vi "pyonpyon2.vi"() -> ()   [LabVIEW 2013]
uses:
  impl/pp2_CTL_SessionInfo.ctl
  impl/pp2_CTL_StateInfo.ctl
  impl/pp2_CTL_State.ctl
  impl/pp2_Trial.ctl
  impl/pp2_CTL_TrialType.ctl
  labolabo2/waveforms/WFTypes.ctl
  impl/pp2_CTL_SessionParamDynamic.ctl
  impl/pp2_CTL_DaqConfig.ctl
  <vilib>/userdefined/High Color/IMAQdx.ctl
  <vilib>/sound2/lvsound2.llb/Sound Output Task ID.ctl
  impl/pp2_CTL_Trial.ctl
  labolabo2/array/impl/NullArray_I.vi
  <vilib>/Utility/file.llb/Read From Spreadsheet File (string).vi
  <vilib>/Utility/file.llb/Write To Spreadsheet File (string).vi
  labolabo2/array/impl/ArrayFirst_S.vi
panel:
  in  "Trial Types Control":enum32{"Trial Types Control"}(tab)
  out "Trial Types File Path":path
  in  "Save Trial Types":bool
  in  "Load Trial Types":bool
  out "Trial Types Valid":bool=TRUE
  in  "Trial Types":T1[](array[typedef])=[{"Trial Type Number"=1, "Trial Type"=enum."GO", "Trial Weight"=1, "Shock (mA)"=-1.0, "Duration (ms)"=250.0, "Sound Type"=enum."04 FM Sweep", "Stim P1"=2000.0, "Stim P2"=4000.0, "Stim P3"=0.0, "Stim P4"=0.0}, {"Trial Type Number"=2, "Trial Type"=enum."NOGO", "Trial Weight"=1, "Shock (mA)"=-1.0, "Duration (ms)"=250.0, "Sound Type"=enum."04 FM Sweep", "Stim P1"=4000.0, "Stim P2"=2000.0, "Stim P3"=0.0, "Stim P4"=0.0}] {"Shock (mA)" min=-1.0 max=5.0; "Trial Weight" step=1; "Duration (ms)" min=0.0 max=1.0; "Trial Type Number" min=1 step=1}
  in  "Session List Control":enum32{"Session List Control"}(tab)
  out "Session List File Path":path=path "E:/Data/SPP.Coulb1/SPP027/ppSessList.141015.1622.tsv"
  in  "Load Session List":bool
  in  "Save Session List":bool
  in  "Generate Session List":bool
  in  "Total Trials":i32=60 min=3 step=1
  in  "Pseudo-Gellerman Start":i32=2 min=2
  out "Session List Valid":bool=TRUE
  out "Session list display":string[][](table)
  in  "Session List Hidden":u8[](array[numeric]) min=1 step=1
  in  "Daq config":T4={"Sound AO"="Dev2/ao0", "Shock intesity AO"="Dev2/ao1", "Code_LED DO"="Dev2/port1:2", "Switch DI"="Dev2/port0/line0:1", "Webcam"="cam9", "Sound AO task"="", "Sound card task"=0, "Shock intensity AO task"="", "Code_LED DO task"="", "Switch DI task"="", "AO <=> Sound card"=FALSE, "Sound card"=0, "sample rate"=8000.0, "Variable shock"=FALSE, "Webcam on"=TRUE, "Tone gate PFI"="/Dev2/PFI1", "Waveform memo"={"t0"=timestamp(0 s since 1904-01-01), "dt"=1.0, "Y"=[]}} {"sample rate" min=8000.0; "Sound card task" format="%.0x"}
  out "Image":T7(plugin-control)
  in  "Session param (dynamic)":T8={"Def M shock (mA)"=400.0, "Def F shock (mA)"=0.0, "Def M shock +/-"=4, "Def F shock +/-"=4} {"Def F shock +/-" min=0 step=1; "Def M shock +/-" min=0 step=1}
  in  "stop":bool
  in  "Pause":bool
  out "State info":T9={"Curr  tr"=0, "Curr (ms)"=0, "Cum (ms)"=0, "Run loop diff"=0, "Tone countdown (ms)"=0, "Countdown (ms)"=0, "Curr State"=enum."0 NULL", "Prev State"=enum."1 Habituation", "Null"=FALSE, "Sw"=FALSE, "Tone\nGate"=FALSE, "Stim"=FALSE, "Current DAQ DO Int"=0, "Current Loaded Trial"={"Trial Type Number"=1, "Trial Type"=enum."GO", "Trial Weight"=100, "Shock (mA)"=0.3, "Duration (ms)"=0.25, "Sound Type"=enum."04 FM Sweep", "Stim P1"=4000.0, "Stim P2"=0.0, "Stim P3"=0.0, "Stim P4"=2000.0}, "Next Trial (for display purposes)"={"Trial Type Number"=1, "Trial Type"=enum."GO", "Trial Weight"=100, "Shock (mA)"=0.3, "Duration (ms)"=0.25, "Sound Type"=enum."04 FM Sweep", "Stim P1"=4000.0, "Stim P2"=0.0, "Stim P3"=0.0, "Stim P4"=2000.0}, "Total trials memo"=0, "State start cum memo (ms)"=0, "Last dur jump time memo (ms)"=0, "Last dur shock time memo (ms)"=0, "Tone repeat memo"=0, "Webcam on"=FALSE, "Webcam recording"=TRUE} {"Current DAQ DO Int" format="%b"; "Next Trial (for display purposes)"."Shock (mA)" min=-1.0 max=5.0; "Next Trial (for display purposes)"."Trial Weight" step=1; "Next Trial (for display purposes)"."Duration (ms)" min=0.0 max=1.0; "Next Trial (for display purposes)"."Trial Type Number" min=1 step=1; "Current Loaded Trial"."Shock (mA)" min=-1.0 max=5.0; "Current Loaded Trial"."Trial Weight" step=1; "Current Loaded Trial"."Duration (ms)" min=0.0 max=1.0; "Current Loaded Trial"."Trial Type Number" min=1 step=1}
  in  "Session parameters":T11={"Log File Directory Root"=path "C:/test", "Habit tr0 (s)"=180, "ITI max\n(s)"=25, "ITI min\n(s)"=15, "Tone repeat (ms)"=0, "Jump time\n(s)"=4, "Subject Name"="SPP030", "Run"=FALSE, "Start trial"=0, "Stay \n(s)"=5, "Log File Directory"=path "", "Shock \ndur (s)"=6, "Pre click \n(V)"=1.0, "Click\ndel (s)"=6} {"Click\ndel (s)" min=0 step=1; "Pre click \n(V)" min=0.0 step=1.0; "Shock \ndur (s)" min=0 step=1; "Stay \n(s)" min=0 step=1; "Start trial" step=1; "Jump time\n(s)" min=0 step=1; "Tone repeat (ms)" min=0 step=1; "ITI min\n(s)" min=0 step=1; "ITI max\n(s)" min=0 step=1; "Habit tr0 (s)" min=0 step=1}
  out "Runtime Errors":errorcluster={"status"=FALSE, "code"=-200552, "source"=""}
  in  "Refresh":bool
  out "Session info":T12
  # "Pyonpyon Labview  v2.5 (2014.12 KT) ktakagak@lin-magdeburg.de)"
  # "Code"
  # "Type"
  # "Dur (ms)"
  # "P 1"
  # "P 2"
  # "P 3"
  # "P 4"
  # "Weight"
  # "Shock"
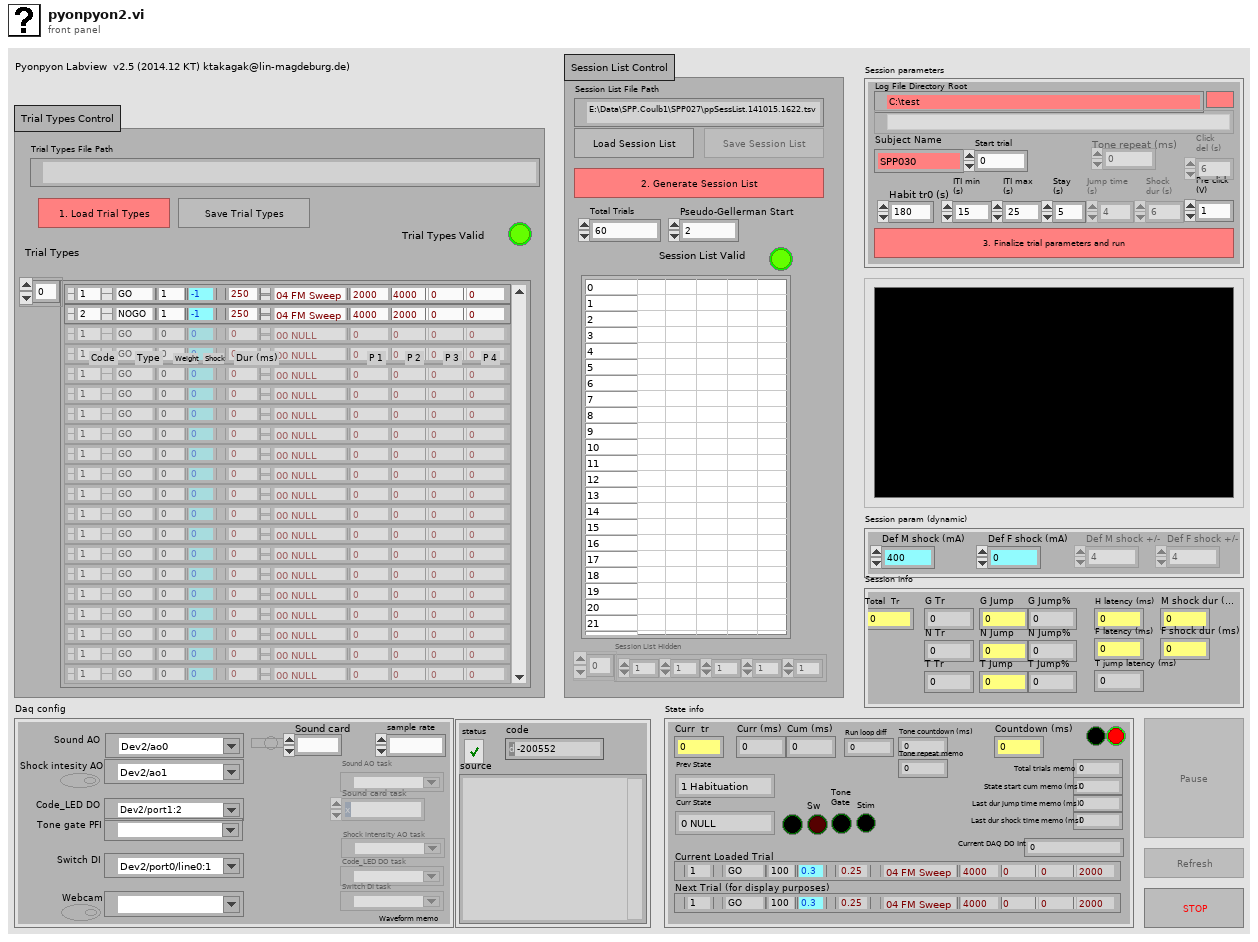
[diagram p1: front panel]
types:
  T1 = typedef "pp2_Trial.ctl" = cluster{"Trial Type Number":u8, "Trial Type":T2, "Trial Weight":u32, "Shock (mA)":dbl, "Duration (ms)":dbl, "Sound Type":T3, "Stim P1":dbl, "Stim P2":dbl, "Stim P3":dbl, "Stim P4":dbl}
  T2 = typedef "pp2_CTL_TrialType.ctl" = enum16{"OFF", "GO", "NOGO", "TEST"}
  T3 = typedef "WFTypes.ctl" = enum16{"00 NULL", "01 DC", "02 Noise", "03 Pure Tone", "04 FM Sweep"}
  T4 = typedef "pp2_CTL_DaqConfig.ctl" = cluster{"Sound AO":tag, "Shock intesity AO":tag, "Code_LED DO":tag, "Switch DI":tag, "Webcam":T5, "Sound AO task":refnum<k21>, "Sound card task":T6, "Shock intensity AO task":refnum<k21>, "Code_LED DO task":refnum<k21>, "Switch DI task":refnum<k21>, "AO <=> Sound card":bool, "Sound card":u32, "sample rate":dbl, "Variable shock":bool, "Webcam on":bool, "Tone gate PFI":tag, "Waveform memo":waveform(dbl)}
  T5 = typedef "IMAQdx.ctl" = refnum<k21>
  T6 = typedef "Sound Output Task ID.ctl" = u32
  T7 = typedef "IMAQ Image.ctl" = refnum<image>
  T8 = typedef "pp2_CTL_SessionParamDynamic.ctl" = cluster{"Def M shock (mA)":dbl, "Def F shock (mA)":dbl, "Def M shock +/-":i32, "Def F shock +/-":i32}
  T9 = typedef "pp2_CTL_StateInfo.ctl" = cluster{"Curr  tr":u16, "Curr (ms)":i64, "Cum (ms)":i64, "Run loop diff":i64, "Tone countdown (ms)":i64, "Countdown (ms)":i64, "Curr State":T10, "Prev State":T10, "Null":bool, "Sw":bool, "Tone\nGate":bool, "Stim":bool, "Current DAQ DO Int":u16, "Current Loaded Trial":T1, "Next Trial (for display purposes)":T1, "Total trials memo":i64, "State start cum memo (ms)":i64, "Last dur jump time memo (ms)":i64, "Last dur shock time memo (ms)":i64, "Tone repeat memo":i64, "Webcam on":bool, "Webcam recording":bool}
  T10 = typedef "pp2_CTL_State.ctl" = enum8{"0 NULL", "1 Habituation", "2 (Load Trial)", "3 Stay Period", "4 Load Audio/Click Delay", "5 GO Trial", "6 GO Jumped", "7 GO Timeout", "8 NOGO Trial", "9 NOGO Jumped", "10 NOGO Timeout", "11 TEST Trial", "12 TEST Jumped", "13 TEST Timeout", "14 Intertrial Interval", "15 Done"}
  T11 = cluster{"Log File Directory Root":path, "Habit tr0 (s)":i32, "ITI max\n(s)":i32, "ITI min\n(s)":i32, "Tone repeat (ms)":i32, "Jump time\n(s)":i32, "Subject Name":string, "Run":bool, "Start trial":u16, "Stay \n(s)":i32, "Log File Directory":path, "Shock \ndur (s)":i32, "Pre click \n(V)":dbl, "Click\ndel (s)":i32}
  T12 = typedef "pp2_CTL_SessionInfo.ctl" = cluster{"Total  Tr":u32, "G Tr":u32, "G Jump":u32, "G Jump%":dbl, "N Tr":u32, "N Jump":u32, "N Jump%":dbl, "T Tr":u32, "T Jump":u32, "T Jump%":dbl, "M shock dur (ms)":dbl, "F shock dur (ms)":dbl, "H latency (ms)":dbl, "F latency (ms)":dbl, "T jump latency (ms)":dbl}
  T13 = enum8{"Enabled", "Disabled", "Disabled and Grayed Out"}
  T14 = typedef "pp2_CTL_Trial.ctl" = cluster{"Trial Type Number":i16, "Trial Type":T2, "Trial Weight":u32, "Shock (mA)":dbl, "Duration (ms)":dbl, "Sound Type":T3, "Stim P1":dbl, "Stim P2":dbl, "Stim P3":dbl, "Stim P4":dbl}
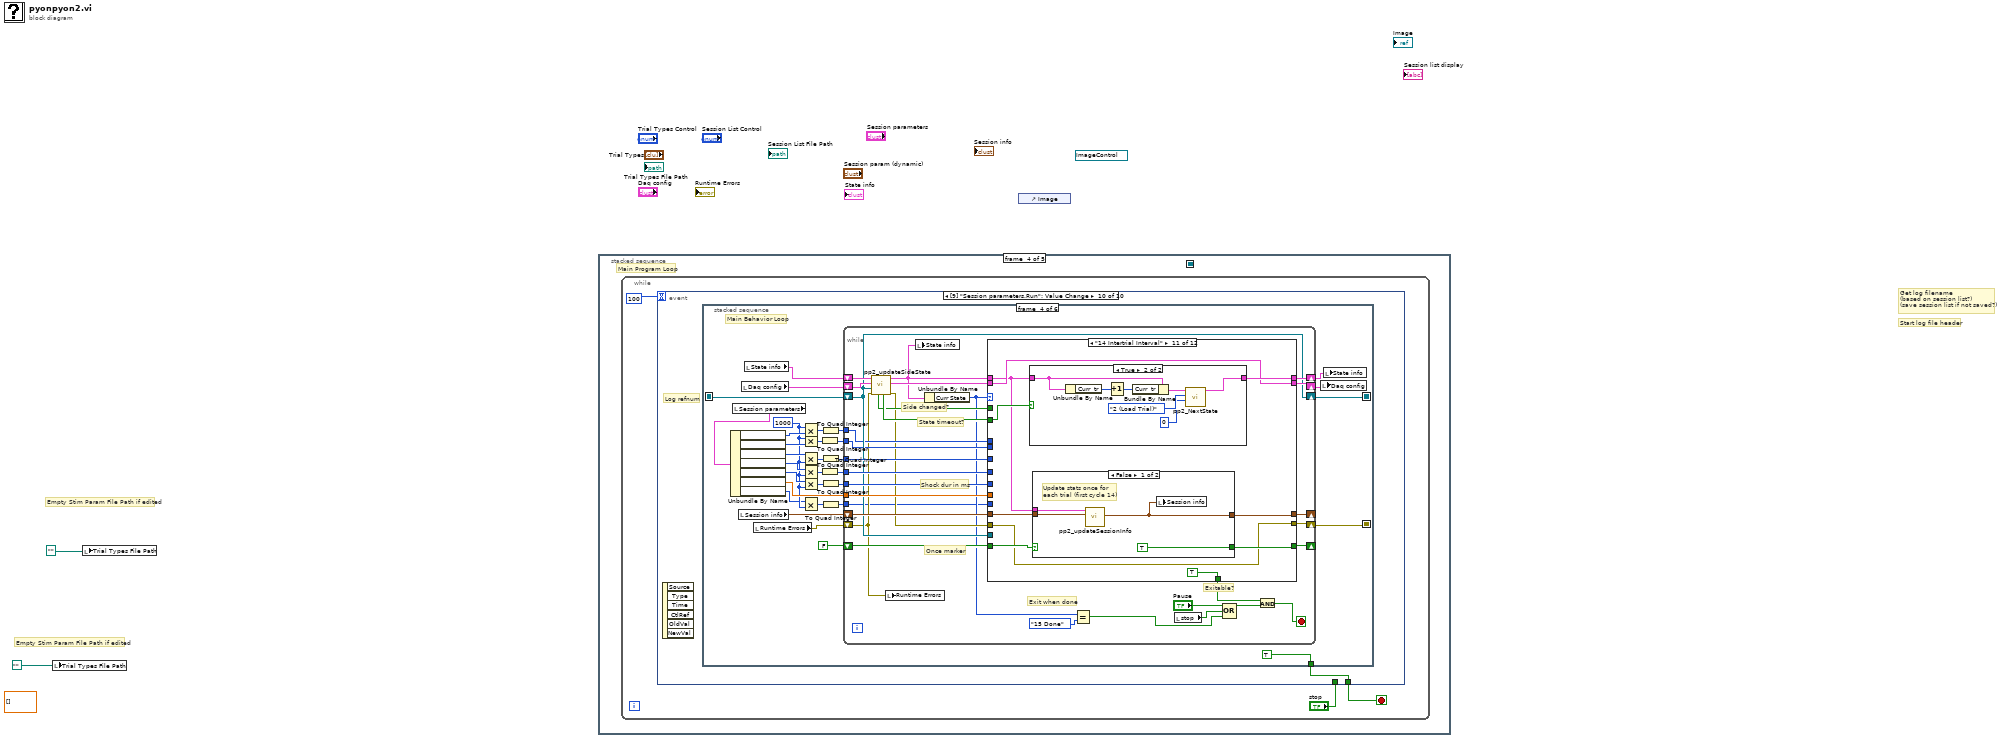
[diagram p0: block diagram]
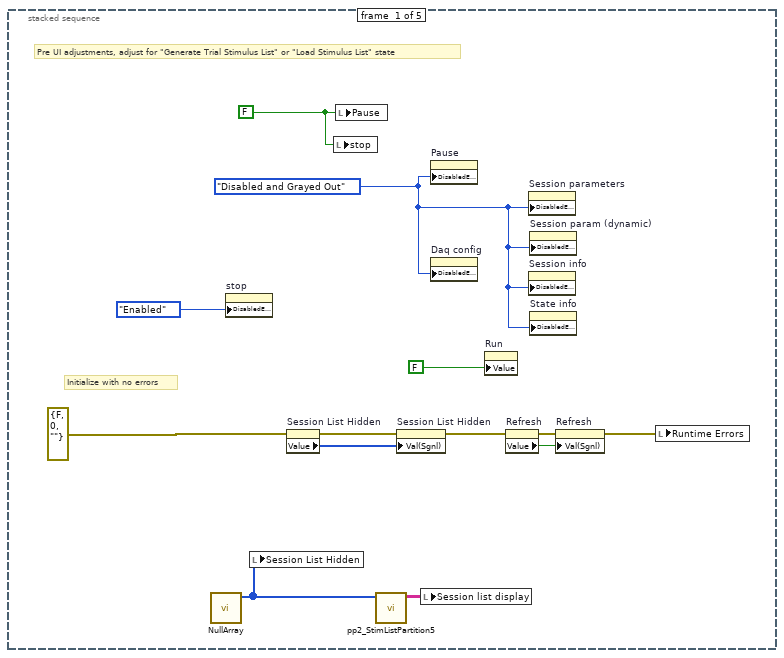
[diagram p2: hidden frame]
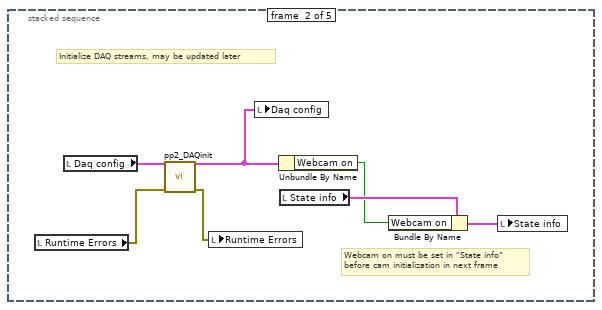
[diagram p3: hidden frame]
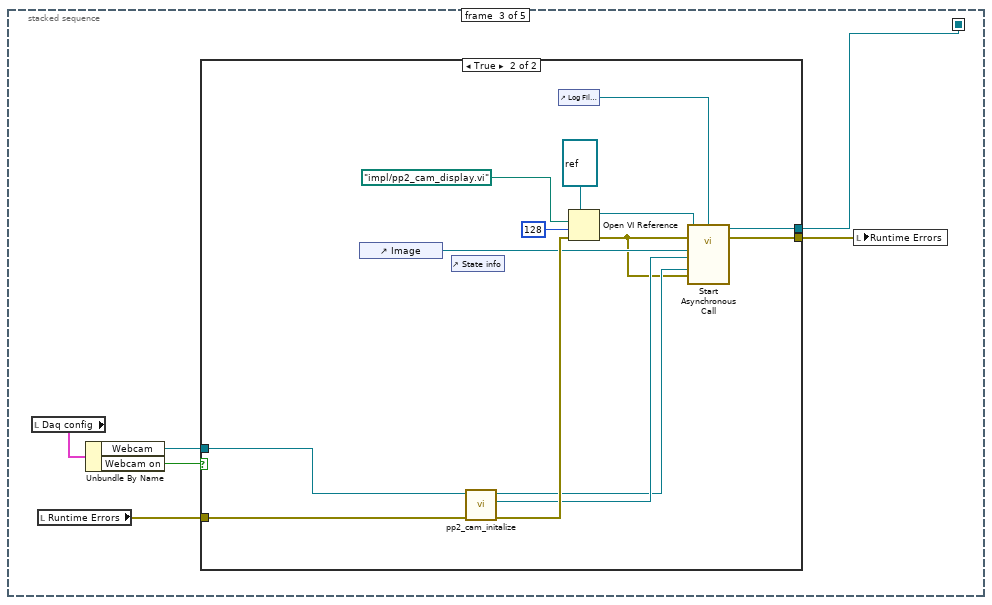
[diagram p4: hidden frame]
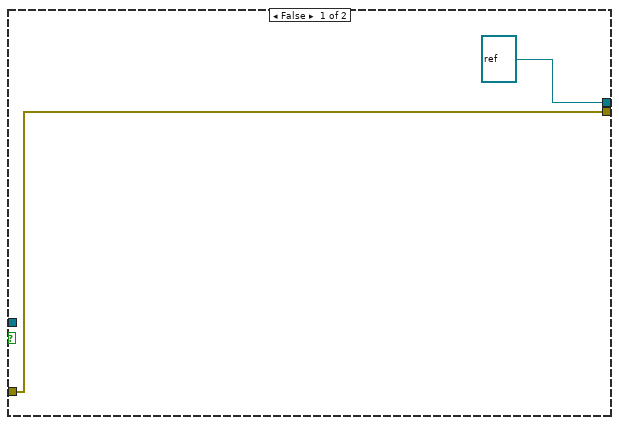
[diagram p5: hidden frame]
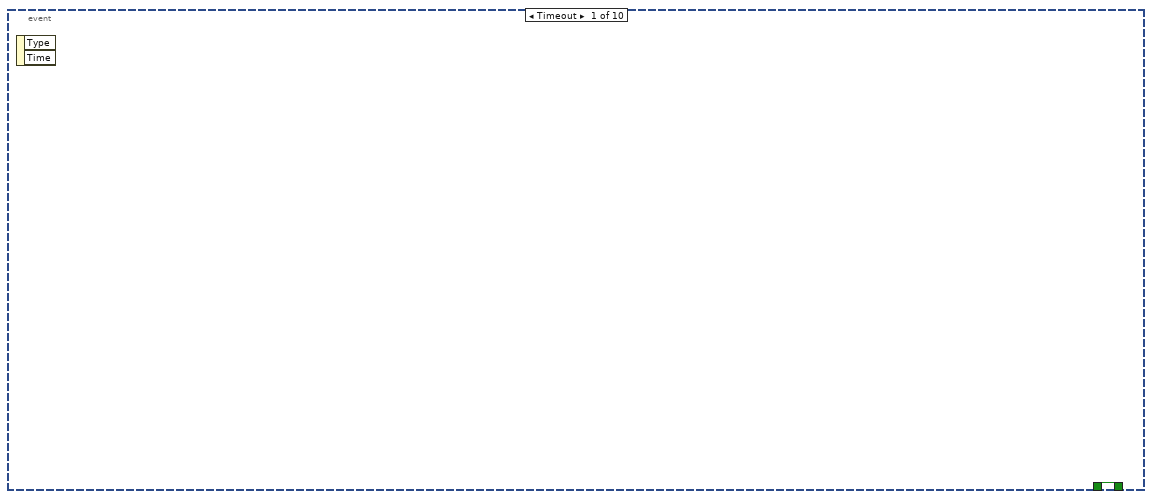
[diagram p6: hidden frame]
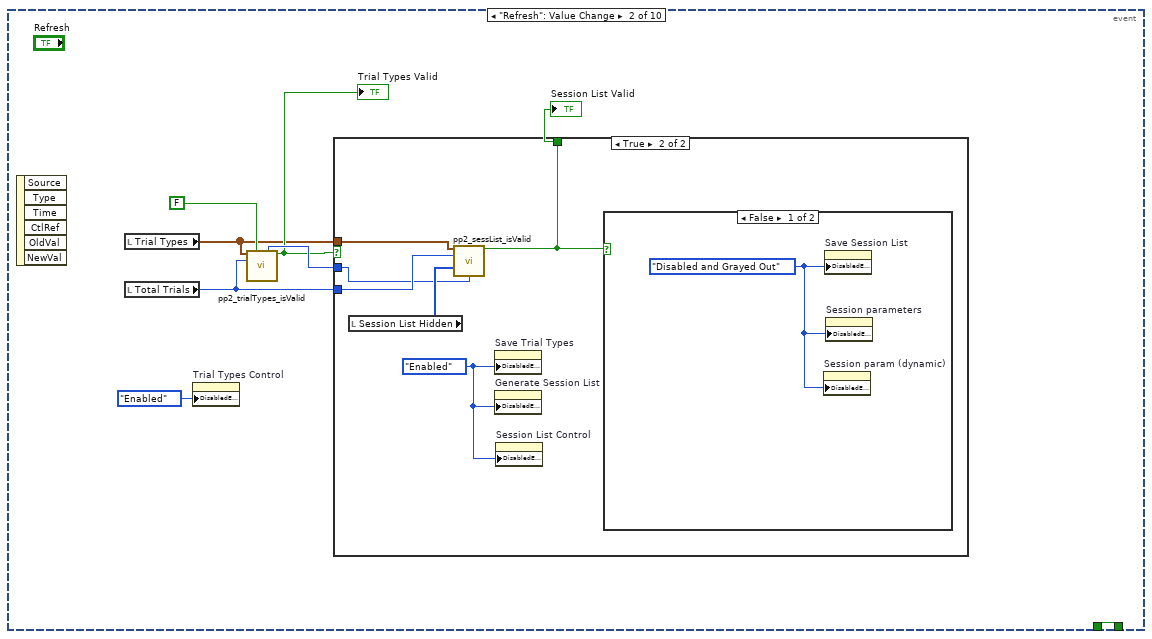
[diagram p7: hidden frame]
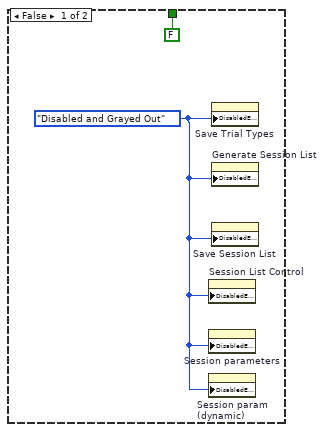
[diagram p8: hidden frame]
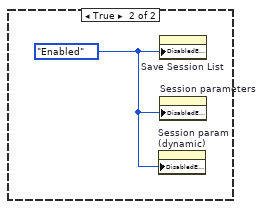
[diagram p9: hidden frame]
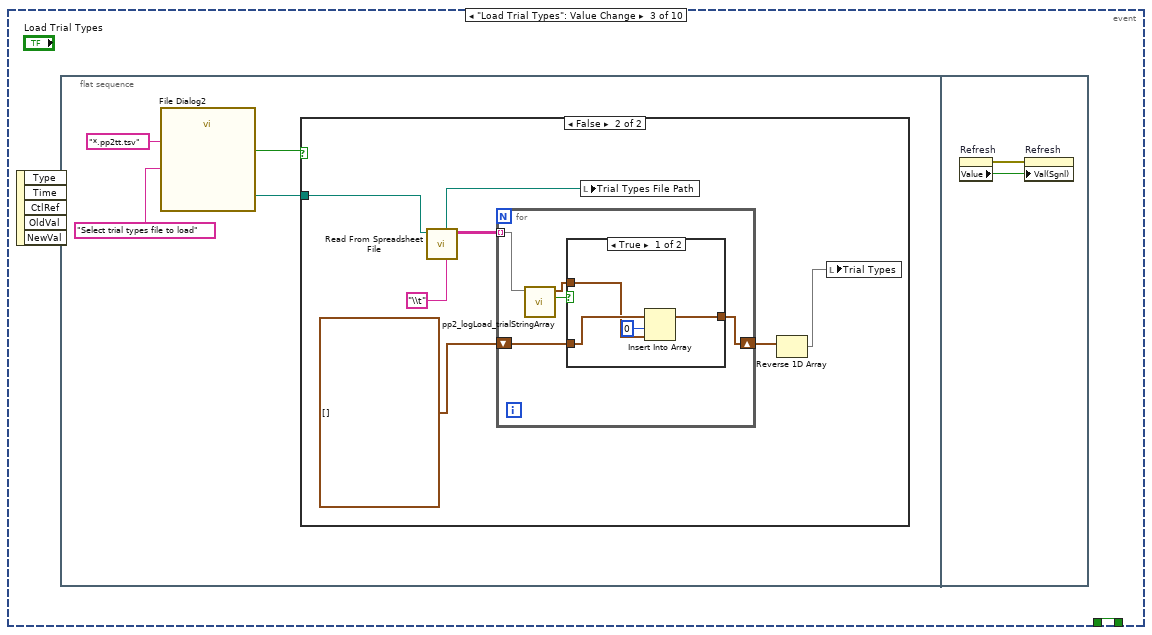
[diagram p10: hidden frame]
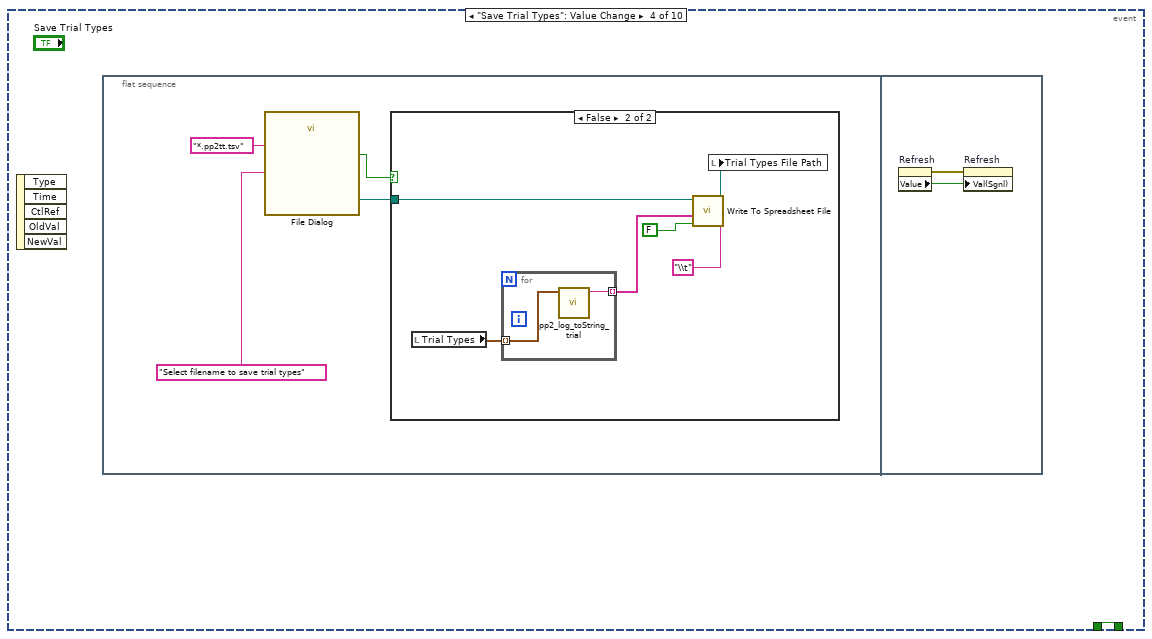
[diagram p13: hidden frame]
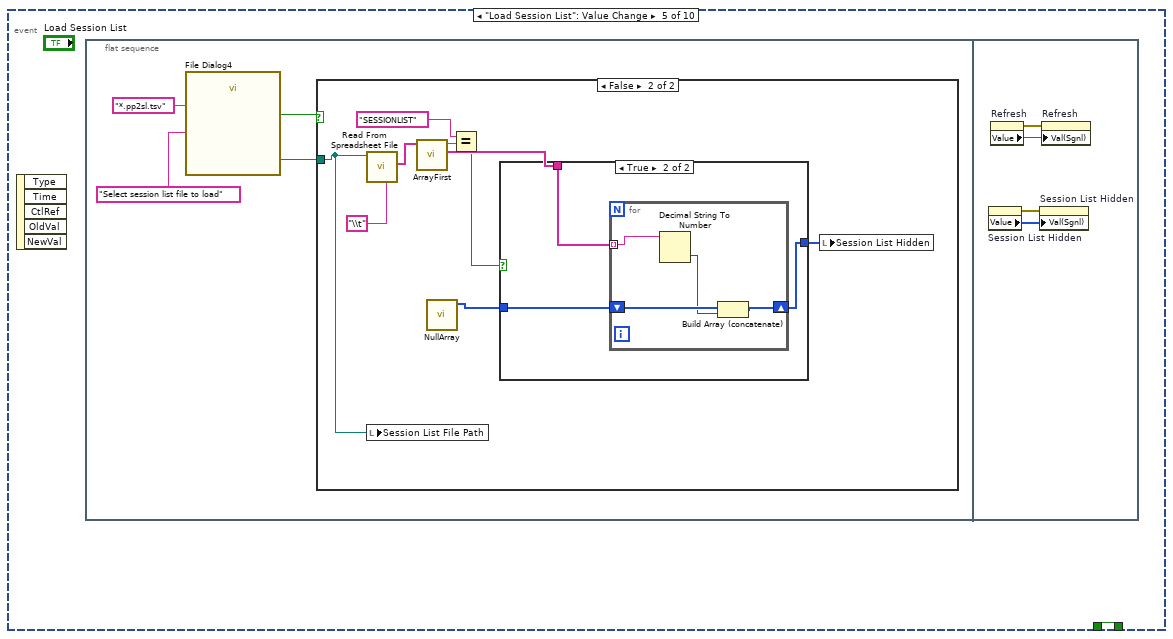
[diagram p15: hidden frame]
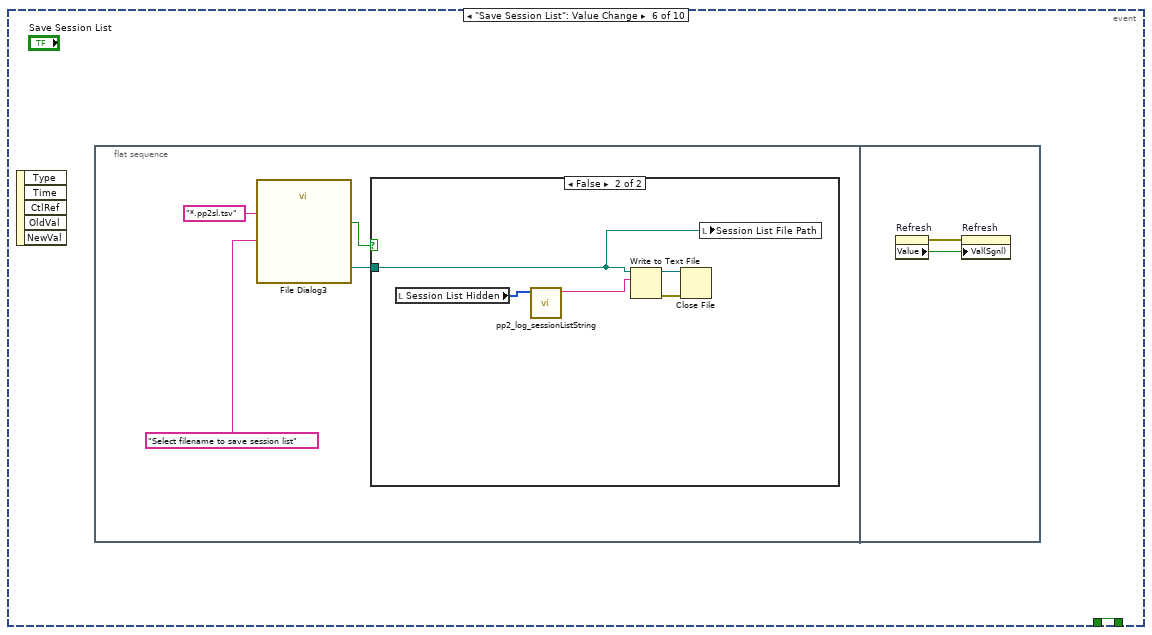
[diagram p18: hidden frame]
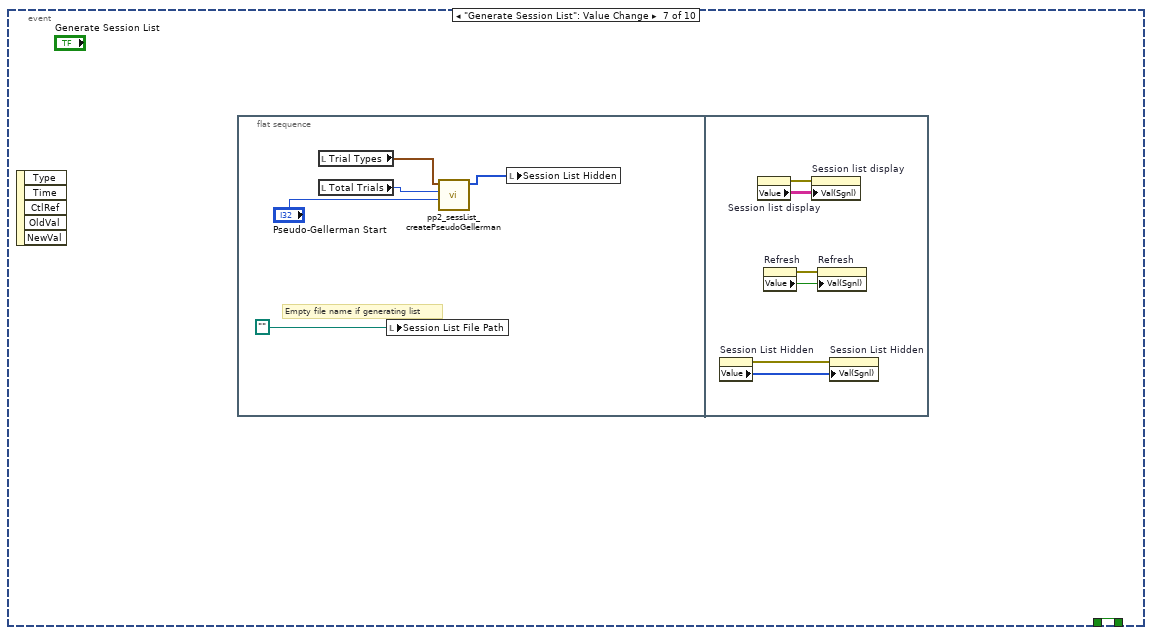
[diagram p20: hidden frame]
diagram:
  (unwired) refnum<vi> refnum ("Image")
  (unwired) dbl[][] []
  # "Start log file header"
  # "Get log filename\n(based on session list?)\n(save session list if not saved?)"
  # "Empty Stim Param File Path if edited"
  # "Empty Stim Param File Path if edited"
  n1 = local write "Trial Types File Path"(path "") -> ()
  n2 = local write "Trial Types File Path"(path "") -> ()
  n3 = stacked-sequence {
    seq-local: [_ _ w23 _ _] -> [_ _ _ _ w633]
    frame #0 {
      w15 = FALSE
      w6 = T13."Disabled and Grayed Out" ("Disabled")
      # "Initialize with no errors"
      # "Pre UI adjustments, adjust for \"Generate Trial Stimulus List\" or \"Load Stimulus List\" state"
      n4 = call-poly "NullArray.vi"() -> ("Null Array"=w5:i32[])  [unwired: 11 in]
      n5 = property on="stop" class="Bool (strict)"("DisabledEnum"=T13."Enabled" ("Disabled")) -> ()  [unwired: 2 in, 2 out]
      n6 = local write "Session List Hidden"(w5) -> ()
      n7 = property on="Session List Hidden" class="Arr (strict)"(error in=errorcluster {"status"=FALSE, "code"=0, "source"=""} ("error in (no error)")) -> (error out=w12:errorcluster, "Value"=w11:u8[])  [unwired: 1 in, 1 out]
      n8 = local write "stop"(w15) -> ()
      n9 = local write "Pause"(w15) -> ()
      n10 = call "pp2_StimListPartition5.vi"("Session List (Hidden variable)"=w5) -> ("Session list display"=w4:string[][])  [unwired: 9 in]
      n11 = property on="Session List Hidden" class="Arr (strict)"(error in=w12, "Val(Sgnl)"=w11) -> (error out=w9:errorcluster)  [unwired: 1 in, 1 out]
      n12 = local write "Session list display"(w4) -> ()
      n13 = property on="Pause" class="Bool (strict)"("DisabledEnum"=w6) -> ()  [unwired: 2 in, 2 out]
      n14 = property on="Daq config" class="Clust (strict)"("DisabledEnum"=w6) -> ()  [unwired: 2 in, 2 out]
      n15 = property on="Run" class="Bool (strict)"("Value"=FALSE) -> ()  [unwired: 2 in, 2 out]
      n16 = property on="Refresh" class="Bool (strict)"(error in=w9) -> (error out=w8:errorcluster, "Value"=w10:bool)  [unwired: 1 in, 1 out]
      n17 = property on="Session parameters" class="Clust (strict)"("DisabledEnum"=w6) -> ()  [unwired: 2 in, 2 out]
      n18 = property on="Session info" class="Clust (strict)"("DisabledEnum"=w6) -> ()  [unwired: 2 in, 2 out]
      n19 = property on="Session param (dynamic)" class="Clust (strict)"("DisabledEnum"=w6) -> ()  [unwired: 2 in, 2 out]
      n20 = property on="State info" class="Clust (strict)"("DisabledEnum"=w6) -> ()  [unwired: 2 in, 2 out]
      n21 = property on="Refresh" class="Bool (strict)"(error in=w8, "Val(Sgnl)"=w10) -> (error out=w7:errorcluster)  [unwired: 1 in, 1 out]
      n22 = local write "Runtime Errors"(w7) -> ()
    }
    frame #1 {
      # "Webcam on must be set in \"State info\"\nbefore cam initialization in next frame"
      # "Initialize DAQ streams, may be updated later"
      n23 = local read "Runtime Errors"() -> (w17:errorcluster)
      n24 = local read "Daq config"() -> (w22:T4)
      n25 = call "pp2_DAQinit.vi"("error in (no error)"=w17, "Daq config in"=w22) -> ("error out"=w16:errorcluster, "Daq config out"=w21:T4)  [unwired: 8 in]
      n26 = local write "Runtime Errors"(w16) -> ()
      n27 = local write "Daq config"(w21) -> ()
      n28 = Unbundle By Name(w21) -> ("Webcam on"=w19:bool)
      n29 = local read "State info"() -> (w20:T9)
      n30 = Bundle By Name(cluster=w20, "Webcam on"=w19) -> (w18:T9)
      n31 = local write "State info"(w18) -> ()
    }
    frame #2 {
      n32 = local read "Daq config"() -> (w26:T4)
      n33 = local read "Runtime Errors"() -> (w27:errorcluster)
      n34 = Unbundle By Name(w26) -> ("Webcam"=w28:T5, "Webcam on"=w25:bool)
      n35 = case shown="True" w25 {
        tunnel: w28 -> [_ w44]
        tunnel: w27 -> [w30 w43]
        tunnel: [w30 w32] -> w24
        tunnel: [refnum<vi> refnum ("type specifier VI Refnum (for type only)") w31] -> w23
        frame False {
        }
        frame True {
          n36 = control-ref of="Image"() -> (w38:refnum<vi>)
          n37 = control-ref of="State info"() -> ()  [unwired: 1 out]
          n38 = call "pp2_cam_initalize.vi"("error in"=w43, "Camera"=w44) -> ("error out"=w41:errorcluster, "Image memory"=w37:T7, "Session Out"=w36:T5)  [unwired: 7 in]
          n39 = control-ref of="Log File Directory"() -> (w39:refnum<vi>)
          n40 = Open VI Reference(type specifier VI Refnum (for type only)=refnum<vi> refnum, vi path=path "impl/pp2_cam_display.vi", options=128, error in (no error)=w41) -> (vi reference=w33:refnum<vi>, error out=w35:errorcluster)  [unwired: 2 in]
          n41 = call-by-ref "Start Asynchronous Call"(reference=w33, error in=w35, "Image Ctl Refnum"=w38, "Log File Directory"=w39, "Image Memory"=w37, "Webcam Session In"=w36, "error in"=w35) -> (reference out=w31:refnum<vi>, error out=w32:errorcluster)  [unwired: 10 in, 1 out]
        }
      }
      n42 = local write "Runtime Errors"(w24) -> ()
    }
    frame #3 {
      # "Main Program Loop"
      n43 = while {
        stop <- w47 stop-if-true
        n44 = event shown="[9] \"Session parameters.Run\": Value Change" {
          selector: _ -> [_ _ _ _ _ _ _ _ _ _]
          dyn-events: _ -> [_ _ _ _ _ _ _ _ _ _]
          timeout: u32 100 ("milliseconds to wait") -> [_ _ _ _ _ _ _ _ _ _]
          tunnel: [w48 w56 w67 w91 w106 w132 w144 w156 w160 w184] -> w47
          tunnel: "stop" -> [w48 w56 w67 w91 w106 w132 w144 w156 w160 _]
          event Timeout {
            n45 = event-data() -> ()  [unwired: 1 in, 2 out]
          }
          event "Refresh": Value Change {
            n46 = event-data() -> ()  [unwired: 1 in, 6 out]
            n47 = local read "Trial Types"() -> (w51:T1[])
            n48 = local read "Total Trials"() -> (w54:i32)
            n49 = property on="Trial Types Control" class="TabCtl (strict)"("DisabledEnum"=T13."Enabled" ("Disabled")) -> ()  [unwired: 2 in, 2 out]
            n50 = call "pp2_trialTypes_isValid.vi"("Trial Types In"=w51, "Throw Error"=FALSE, "Total Trials"=w54) -> ("Trial Replication Factor"=w55:i32, "Paradigm Valid?"=w52:bool)  [unwired: 7 in, 4 out]
            "Trial Types Valid" <- w52
            n51 = case shown="True" w52 {
              tunnel: w55 -> [_ w61]
              tunnel: w54 -> [_ w64]
              tunnel: w51 -> [_ w63]
              tunnel: [FALSE ("Session List Valid?") w60] -> w50
              frame False {
                w57 = T13."Disabled and Grayed Out" ("Disabled")
                n52 = property on="Session List Control" class="TabCtl (strict)"("DisabledEnum"=w57) -> ()  [unwired: 2 in, 2 out]
                n53 = property on="Session parameters" class="Clust (strict)"("DisabledEnum"=w57) -> ()  [unwired: 2 in, 2 out]
                n54 = property on="Session param (dynamic)" class="Clust (strict)"("DisabledEnum"=w57) -> ()  [unwired: 2 in, 2 out]
                n55 = property on="Save Trial Types" class="Bool"("DisabledEnum"=w57) -> ()  [unwired: 2 in, 2 out]
                n56 = property on="Generate Session List" class="Bool"("DisabledEnum"=w57) -> ()  [unwired: 2 in, 2 out]
                n57 = property on="Save Session List" class="Bool"("DisabledEnum"=w57) -> ()  [unwired: 2 in, 2 out]
              }
              frame True {
                w59 = T13."Enabled" ("Disabled")
                n58 = local read "Session List Hidden"() -> (w62:u8[])
                n59 = call "pp2_sessList_isValid.vi"("Trial Types In"=w63, "Total Trials"=w64, "Session List"=w62, "Trial Replication Factor"=w61) -> ("Session List Valid?"=w60:bool)  [unwired: 11 in]
                n60 = property on="Save Trial Types" class="Bool"("DisabledEnum"=w59) -> ()  [unwired: 2 in, 2 out]
                n61 = property on="Generate Session List" class="Bool"("DisabledEnum"=w59) -> ()  [unwired: 2 in, 2 out]
                n62 = property on="Session List Control" class="TabCtl (strict)"("DisabledEnum"=w59) -> ()  [unwired: 2 in, 2 out]
                n63 = case shown="False" w60 {
                  frame False {
                    w65 = T13."Disabled and Grayed Out" ("Disabled")
                    n64 = property on="Session param (dynamic)" class="Clust (strict)"("DisabledEnum"=w65) -> ()  [unwired: 2 in, 2 out]
                    n65 = property on="Save Session List" class="Bool"("DisabledEnum"=w65) -> ()  [unwired: 2 in, 2 out]
                    n66 = property on="Session parameters" class="Clust (strict)"("DisabledEnum"=w65) -> ()  [unwired: 2 in, 2 out]
                  }
                  frame True {
                    w66 = T13."Enabled" ("Disabled")
                    n67 = property on="Session param (dynamic)" class="Clust (strict)"("DisabledEnum"=w66) -> ()  [unwired: 2 in, 2 out]
                    n68 = property on="Save Session List" class="Bool"("DisabledEnum"=w66) -> ()  [unwired: 2 in, 2 out]
                    n69 = property on="Session parameters" class="Clust (strict)"("DisabledEnum"=w66) -> ()  [unwired: 2 in, 2 out]
                  }
                }
              }
            }
            "Session List Valid" <- w50
          }
          event "Load Trial Types": Value Change {
            n70 = event-data() -> ()  [unwired: 1 in, 5 out]
            n71 = flat-sequence {
              frame #0 {
                n72 = call "File Dialog2"("prompt"="Select trial types file to load", "pattern (all files)"="*.pp2tt.tsv") -> ("selected path"=w69:path, "cancelled"=w68:bool)  [unwired: 10 in, 2 out]
                n73 = case shown="False" w68 {
                  tunnel: w69 -> [_ w72]
                  frame True {
                  }
                  frame False {
                    n74 = call-poly <vilib>:"Read From Spreadsheet File.vi"("delimiter (\\t)"="\\t" ("delimiter (\\t)"), "file path (dialog if empty)"=w72) -> ("all rows"=w76:string[][], "new file path (Not A Path if cancelled)"=w77:path)  [unwired: 5 in, 3 out]
                    n75 = for {
                      tunnel: w76 -> [w82] mode=indexing
                      shift-right: [w80] -> w74
                      shift-left: T14[] [] -> [w81]
                      n76 = call "pp2_logLoad_trialStringArray.vi"("Input string array"=w82) -> ("Was TRIAL?"=w79:bool, "Trial in"=w83:T14)  [unwired: 7 in]
                      n77 = case shown="True" w79 {
                        tunnel: w83 -> [w86 _]
                        tunnel: w81 -> [w87 w88]
                        tunnel: [w84 w88] -> w80
                        frame True {
                          n78 = Insert Into Array(array=w87, index=0, new element=w86) -> (w84:T14[])
                        }
                        frame False {
                        }
                      }
                    }
                    n79 = local write "Trial Types File Path"(w77) -> ()
                    n80 = Reverse 1D Array(array=w74) -> (reversed array=w73:T14[])
                    n81 = local write "Trial Types"(w73) -> ()
                  }
                }
              }
              frame #1 {
                n82 = property on="Refresh" class="Bool (strict)"() -> (error out=w90:errorcluster, "Value"=w89:bool)  [unwired: 2 in, 1 out]
                n83 = property on="Refresh" class="Bool (strict)"(error in=w90, "Val(Sgnl)"=w89) -> ()  [unwired: 1 in, 2 out]
              }
            }
          }
          event "Save Trial Types": Value Change {
            n84 = event-data() -> ()  [unwired: 1 in, 5 out]
            n85 = flat-sequence {
              frame #0 {
                n86 = call "File Dialog"("prompt"="Select filename to save trial types", "pattern (all files)"="*.pp2tt.tsv") -> ("selected path"=w95:path, "cancelled"=w94:bool)  [unwired: 10 in, 2 out]
                n87 = case shown="False" w94 {
                  tunnel: w95 -> [_ w96]
                  frame True {
                  }
                  frame False {
                    n88 = local read "Trial Types"() -> (w99:T1[])
                    n89 = for {
                      tunnel: w99 -> [w103] mode=indexing
                      tunnel: [w102] -> w98 mode=indexing
                      n90 = call "pp2_log_toString_trial.vi"("Trial in"=w103) -> ("spreadsheet string"=w102:string)  [unwired: 10 in]
                    }
                    n91 = call-poly <vilib>:"Write To Spreadsheet File.vi"("delimiter (\\t)"="\\t" ("delimiter (\\t)"), "append to file? (new file:F)"=FALSE, "1D data"=w98, "file path (dialog if empty)"=w96) -> ("new file path (Not A Path if cancelled)"=w100:path)  [unwired: 4 in]
                    n92 = local write "Trial Types File Path"(w100) -> ()
                  }
                }
              }
              frame #1 {
                n93 = property on="Refresh" class="Bool (strict)"() -> (error out=w105:errorcluster, "Value"=w104:bool)  [unwired: 2 in, 1 out]
                n94 = property on="Refresh" class="Bool (strict)"(error in=w105, "Val(Sgnl)"=w104) -> ()  [unwired: 1 in, 2 out]
              }
            }
          }
          event "Load Session List": Value Change {
            n95 = event-data() -> ()  [unwired: 1 in, 5 out]
            n96 = flat-sequence {
              frame #0 {
                n97 = call "File Dialog4"("prompt"="Select session list file to load", "pattern (all files)"="*.pp2sl.tsv") -> ("selected path"=w108:path, "cancelled"=w107:bool)  [unwired: 10 in, 2 out]
                n98 = case shown="False" w107 {
                  tunnel: w108 -> [_ w114]
                  frame True {
                  }
                  frame False {
                    n99 = call-poly <vilib>:"Read From Spreadsheet File.vi"("delimiter (\\t)"="\\t" ("delimiter (\\t)"), "file path (dialog if empty)"=w114) -> ("first row"=w118:string[])  [unwired: 5 in, 4 out]
                    n100 = local write "Session List File Path"(w114) -> ()
                    n101 = call-poly "ArrayFirst.vi"("1D Array In"=w118) -> ("Rest of Array"=w115:string[], "First Element"=w117:string)  [unwired: 9 in]
                    n102 = call-poly "NullArray.vi"() -> ("Null Array"=w111:i32[])  [unwired: 11 in]
                    n103 = Equal?(x="SESSIONLIST", y=w117) -> (x = y?=w113:bool)
                    n104 = case shown="True" w113 {
                      tunnel: w115 -> [_ w123]
                      tunnel: [w120 w122] -> w112
                      tunnel: w111 -> [w120 w121]
                      frame False {
                      }
                      frame True {
                        n105 = for {
                          shift-right: [w127] -> w122
                          shift-left: w121 -> [w126]
                          tunnel: w123 -> [w125] mode=indexing
                          n106 = Decimal String To Number(string=w125) -> (number=w124:i32)  [unwired: 2 in, 1 out]
                          n107 = Build Array (concatenate)(w126, w124) -> (w127:i32[])
                        }
                      }
                    }
                    n108 = local write "Session List Hidden"(w112) -> ()
                  }
                }
              }
              frame #1 {
                n109 = property on="Session List Hidden" class="Arr (strict)"() -> (error out=w128:errorcluster, "Value"=w129:u8[])  [unwired: 2 in, 1 out]
                n110 = property on="Refresh" class="Bool (strict)"() -> (error out=w131:errorcluster, "Value"=w130:bool)  [unwired: 2 in, 1 out]
                n111 = property on="Session List Hidden" class="Arr (strict)"(error in=w128, "Val(Sgnl)"=w129) -> ()  [unwired: 1 in, 2 out]
                n112 = property on="Refresh" class="Bool (strict)"(error in=w131, "Val(Sgnl)"=w130) -> ()  [unwired: 1 in, 2 out]
              }
            }
          }
          event "Save Session List": Value Change {
            n113 = event-data() -> ()  [unwired: 1 in, 5 out]
            n114 = flat-sequence {
              frame #0 {
                n115 = call "File Dialog3"("prompt"="Select filename to save session list", "pattern (all files)"="*.pp2sl.tsv") -> ("selected path"=w136:path, "cancelled"=w135:bool)  [unwired: 10 in, 2 out]
                n116 = case shown="False" w135 {
                  tunnel: w136 -> [_ w139]
                  frame True {
                  }
                  frame False {
                    n117 = local read "Session List Hidden"() -> (w141:u8[])
                    n118 = call "pp2_log_sessionListString.vi"("Session List in"=w141) -> ("spreadsheet string"=w140:string)  [unwired: 10 in]
                    n119 = Write to Text File(file (use dialog)=w139, text=w140) -> (refnum out=w137:refnum<file>, error out=w138:errorcluster)  [unwired: 2 in, 1 out]
                    n120 = Close File(refnum=w137, error in=w138) -> ()  [unwired: 2 out]
                    n121 = local write "Session List File Path"(w139) -> ()
                  }
                }
              }
              frame #1 {
                n122 = property on="Refresh" class="Bool (strict)"() -> (error out=w143:errorcluster, "Value"=w142:bool)  [unwired: 2 in, 1 out]
                n123 = property on="Refresh" class="Bool (strict)"(error in=w143, "Val(Sgnl)"=w142) -> ()  [unwired: 1 in, 2 out]
              }
            }
          }
          event "Generate Session List": Value Change {
            n124 = event-data() -> ()  [unwired: 1 in, 5 out]
            n125 = flat-sequence {
              frame #0 {
                # "Empty file name if generating list"
                n126 = local read "Trial Types"() -> (w146:T1[])
                n127 = local read "Total Trials"() -> (w149:i32)
                n128 = local write "Session List File Path"(path "") -> ()
                n129 = call "pp2_sessList_createPseudoGellerman.vi"("Start Num"="Pseudo-Gellerman Start", "Total Trials"=w149, "Trial Types"=w146) -> ("Session List (Cannot Edit)"=w145:i32[])  [unwired: 7 in, 1 out]
                n130 = local write "Session List Hidden"(w145) -> ()
              }
              frame #1 {
                n131 = property on="Session List Hidden" class="Arr (strict)"() -> (error out=w151:errorcluster, "Value"=w150:u8[])  [unwired: 2 in, 1 out]
                n132 = property on="Session list display" class="Tbl (strict)"() -> (error out=w153:errorcluster, "Value"=w152:string[][])  [unwired: 2 in, 1 out]
                n133 = property on="Refresh" class="Bool (strict)"() -> (error out=w155:errorcluster, "Value"=w154:bool)  [unwired: 2 in, 1 out]
                n134 = property on="Session list display" class="Tbl (strict)"(error in=w153, "Val(Sgnl)"=w152) -> ()  [unwired: 1 in, 2 out]
                n135 = property on="Refresh" class="Bool (strict)"(error in=w155, "Val(Sgnl)"=w154) -> ()  [unwired: 1 in, 2 out]
                n136 = property on="Session List Hidden" class="Arr (strict)"(error in=w151, "Val(Sgnl)"=w150) -> ()  [unwired: 1 in, 2 out]
              }
            }
          }
          event "Total Trials": Value Change {
            n137 = event-data() -> ()  [unwired: 1 in, 6 out]
            n138 = flat-sequence {
              tunnel: "Total Trials" -> [_]
              frame #0 {
              }
              frame #1 {
                n139 = property on="Refresh" class="Bool (strict)"() -> (error out=w158:errorcluster, "Value"=w159:bool)  [unwired: 2 in, 1 out]
                n140 = property on="Refresh" class="Bool (strict)"(error in=w158, "Val(Sgnl)"=w159) -> ()  [unwired: 1 in, 2 out]
              }
            }
          }
          event "Session List Hidden": Value Change {
            # "Init (r,c)"
            n141 = event-data() -> ()  [unwired: 1 in, 6 out]
            n142 = call "pp2_StimListPartition5.vi"("Session List (Hidden variable)"="Session List Hidden") -> ("Session list display"=w167:string[][])  [unwired: 9 in]
            n143 = local write "Session list display"(w167) -> ()
            n144 = Initialize Array(0, 2 ("dimension size")) -> (w165:i32[])
            n145 = for {
              N: 24 -> [_]
              shift-right: [w172] -> _
              shift-left: w165 -> [w175]
              tunnel: u32 16448250 -> [w171]
              tunnel: [w169] -> w161 mode=indexing
              i -> [w170]
              n146 = Replace Array Subset(array=w175, new element=w170, index=0) -> (w174:i32[])
              n147 = for {
                N: 5 -> [_]
                shift-right: [w181] -> w172
                shift-left: w174 -> [w182]
                tunnel: w170 -> [w180]
                tunnel: w171 -> [w177]
                i -> [w179]
                n148 = Replace Array Subset(array=w182, new element=w179, index=1) -> (w181:i32[])
                n149 = Bundle(w180, w179) -> (w178:cluster{i32, i32})  [unwired: 1 in]
                n150 = property on="Session list display" class="Tbl (strict)"("Active Cell"=w178, "Cell BG Color"=w177) -> ()  [unwired: 2 in, 2 out]
              }
              n151 = Number To Decimal String(number=w170) -> (decimal integer string=w169:string)  [unwired: 1 in]
            }
            n152 = property on="Session list display" class="Tbl (strict)"("Row Headers[]"=w161) -> ()  [unwired: 2 in, 2 out]
          }
          event "Session parameters.Run": Value Change {
            # "Log refnum"
            n153 = event-data() -> ()  [unwired: 1 in, 6 out]
            n154 = stacked-sequence {
              seq-local: [_ _ w236 _ _ _] -> [_ _ _ w252 _ _]
              seq-local: [_ _ _ w283 _ _] -> [_ _ _ _ w628 _]
              seq-local: [_ _ _ w264 _ _] -> [_ _ _ _ _ _]
              tunnel: [_ _ _ TRUE _ _] -> w184
              frame #0 {
                w185 = T13."Disabled and Grayed Out" ("Disabled")
                # "Confirm if starting with nonzero trial"
                # "GUI Adjustments (pre)"
                n155 = local read "Session parameters"() -> (w187:T11)
                n156 = Unbundle By Name(w187) -> ("Start trial"=w188:u16)
                n157 = Not Equal To 0?(x=w188) -> (x != 0?=w189:bool)
                n158 = case shown="True" w189 {
                  tunnel: w188 -> [_ w193]
                  tunnel: w187 -> [_ w190]
                  frame False {
                  }
                  frame True {
                    n159 = Number To Decimal String(number=w193) -> (decimal integer string=w194:string)  [unwired: 1 in]
                    n160 = Concatenate Strings("Really start with nonzero trial?: " ("message"), w194) -> (w192:string)
                    n161 = Two Button Dialog(message=w192, 1:"No, start from zero" ("F button name (\"Cancel\")"), 2:"Yes" ("T button name (\"OK\")")) -> (T button?=w191:bool)
                    n162 = case shown="False" w191 {
                      tunnel: w190 -> [w200 _]
                      frame False {
                        n163 = Bundle By Name(cluster=w200, "Start trial"=u16 0) -> (w198:T11)
                        n164 = local write "Session parameters"(w198) -> ()
                      }
                      frame True {
                        # "Just proceed"
                      }
                    }
                  }
                }
                n165 = property on="Trial Types Control" class="TabCtl (strict)"("DisabledEnum"=w185) -> ()  [unwired: 2 in, 2 out]
                n166 = property on="Session List Control" class="TabCtl (strict)"("DisabledEnum"=w185) -> ()  [unwired: 2 in, 2 out]
                n167 = property on="Session parameters" class="Clust (strict)"("DisabledEnum"=w185) -> ()  [unwired: 2 in, 2 out]
                n168 = property on="Pause" class="Bool (strict)"("DisabledEnum"=T13."Enabled" ("Disabled")) -> ()  [unwired: 2 in, 2 out]
              }
              frame #1 {
                # "If webcam is on, start recording"
                # "Reset trial to zero if exceeded total"
                # "If starting from trial zero, clear and habituate, if not, directly to load trial"
                # "Pre-behavior state and statistics adjustments"
                n169 = local read "Session parameters"() -> (w215:T11)
                n170 = Unbundle By Name(w215) -> ("Start trial"=w208:u16, "Habit tr0 (s)"=w210:i32, "Tone repeat (ms)"=w204:i32)  [unwired: 1 out]
                n171 = local read "Session List Hidden"() -> (w206:u8[])
                n172 = Array Size(array=w206) -> (size(s)=w205:i32)
                n173 = Greater Or Equal?(x=w208, y=w205) -> (x >= y?=w209:bool)
                n174 = case shown="True" w209 {
                  tunnel: w208 -> [w216 _]
                  tunnel: [w216 u16 0 ("Curr  tr")] -> w207
                  frame False {
                  }
                  frame True {
                  }
                }
                n175 = Equal To 0?(x=w207) -> (x = 0?=w214:bool)
                n176 = local read "State info"() -> (w203:T9)
                n177 = Unbundle By Name(w203) -> ("Webcam on"=w202:bool)
                n178 = Bundle By Name(cluster=w203, "Curr  tr"=w207, "Curr State"=pp2_CTL_State."1 Habituation", "Prev State"=pp2_CTL_State."0 NULL", "Total trials memo"=w205, "Tone repeat memo"=w204, "Webcam recording"=w202) -> (w211:T9)
                n179 = case shown="True" w214 {
                  tunnel: w211 -> [w220 w235]
                  tunnel: w210 -> [_ w226]
                  tunnel: [w219 w227] -> w201
                  frame False {
                    n180 = call "pp2_NextState.vi"("New state countdown (ms)"=i64 0, "New State"=pp2_CTL_State."2 (Load Trial)", "State In"=w220) -> ("State Out"=w219:T9)  [unwired: 8 in]
                  }
                  frame True {
                    n181 = Tick Count (ms)() -> (millisecond timer value=w234:u32)
                    n182 = local read "Session info"() -> (w222:T12)
                    n183 = To Quad Integer(1:w234) -> (0:w233:i64)
                    n184 = call "pp2_updateSessionInfoCLEAR.vi"("Session info In"=w222) -> ("Session info Out"=w223:T12)  [unwired: 10 in]
                    n185 = Bundle By Name(cluster=w235, "Curr (ms)"=w233, "Cum (ms)"=i64 0) -> (w231:T9)
                    n186 = local write "Session info"(w223) -> ()
                    n187 = To Quad Integer(1:w226) -> (0:w225:i64)
                    n188 = Multiply(x=w225, y=i64 1000) -> (x*y=w228:i64)
                    n189 = call "pp2_NextState.vi"("Actually run (passthrough if off)"=TRUE, "New state countdown (ms)"=w228, "New State"=pp2_CTL_State."1 Habituation", "State In"=w231) -> ("State Out"=w227:T9)  [unwired: 7 in]
                  }
                }
                n190 = local write "State info"(w201) -> ()
              }
              frame #2 {
                # "Initialize log directory"
                n191 = local read "Session parameters"() -> (w246:T11)
                n192 = Unbundle By Name(w246) -> ("Log File Directory Root"=w240:path, "Subject Name"=w243:string)
                n193 = Format Date/Time String(time format string (%c)="\\%y%m%d\\%H%M\\") -> (date/time string=w244:string)  [unwired: 2 in]
                n194 = Concatenate Strings(w243, w244) -> (w238:string)
                n195 = Concatenate Strings(w238, "runLog.pp2") -> (w239:string)
                n196 = Build Path(base path=w240, name or relative path=w238) -> (appended path=w242:path)
                n197 = Build Path(base path=w240, name or relative path=w239) -> ()  [unwired: 1 out]
                n198 = Bundle By Name(cluster=w246, "Log File Directory"=w242) -> (w241:T11)
                n199 = disable-structure shown="Disabled" {
                  disable-tunnel: [w247 _] -> w236
                  frame Disabled {
                    n200 = Build Array("\"TRIAL\"" ("element")) -> (w249:string[])  [unwired: 10 in]
                    n201 = Open/Create/Replace File() -> (refnum out=w247:refnum<file>)  [unwired: 6 in, 2 out]
                    n202 = Array To Spreadsheet String(delimiter (Tab)="\\t", array=w249, 3:"%s" ("format string")) -> ()  [unwired: 1 out]
                  }
                  frame Enabled {
                  }
                }
                n203 = local write "Session parameters"(w241) -> ()
              }
              frame #3 {
                w260 = 1000 ("y")
                # "Main Behavior Loop"
                n204 = local read "Session parameters"() -> (w280:T11)
                n205 = Unbundle By Name(w280) -> ("ITI max\n(s)"=w268:i32, "ITI min\n(s)"=w267:i32, "Stay \n(s)"=w281:i32, "Jump time\n(s)"=w276:i32, "Shock \ndur (s)"=w275:i32, "Pre click \n(V)"=w272:dbl, "Click\ndel (s)"=w259:i32)
                n206 = local read "Session info"() -> (w253:T12)
                n207 = local read "Daq config"() -> (w262:T4)
                n208 = local read "State info"() -> (w254:T9)
                n209 = local read "Runtime Errors"() -> (w263:errorcluster)
                n210 = Multiply(x=w260, y=w268) -> (x*y=w270:i32)
                n211 = Multiply(x=w260, y=w267) -> (x*y=w269:i32)
                n212 = Multiply(x=w281, y=w260) -> (x*y=w282:i32)
                n213 = Multiply(x=w276, y=w260) -> (x*y=w278:i32)
                n214 = Multiply(x=w275, y=w260) -> (x*y=w277:i32)
                n215 = Multiply(x=w259, y=w260) -> (x*y=w258:i32)
                n216 = To Quad Integer(1:w269) -> (0:w265:i64)
                n217 = To Quad Integer(1:w278) -> (0:w274:i64)
                n218 = To Quad Integer(1:w270) -> (0:w266:i64)
                n219 = To Quad Integer(1:w282) -> (0:w279:i64)
                n220 = To Quad Integer(1:w277) -> (0:w273:i64)
                n221 = To Quad Integer(1:w258) -> (0:w257:i64)
                n222 = while {
                  shift-right: [w310] -> w256
                  shift-left: w254 -> [w309]
                  shift-right: [w306] -> _
                  shift-left: w253 -> [w314]
                  shift-right: [w307] -> w255
                  shift-left: w262 -> [w313]
                  shift-right: [w300] -> w283
                  shift-left: w252 -> [w300]
                  tunnel: w279 -> [w305]
                  tunnel: w274 -> [w304]
                  tunnel: w273 -> [w303]
                  tunnel: w272 -> [w302]
                  shift-right: [w301] -> w264
                  shift-left: w263 -> [w292]
                  shift-right: [w298] -> _
                  shift-left: FALSE -> [w299]
                  tunnel: w266 -> [w297]
                  tunnel: w265 -> [w296]
                  tunnel: w257 -> [w284]
                  stop <- w288 stop-if-true
                  # "Shock dur in ms"
                  # "Exit when done"
                  # "Exitable?"
                  # "Once marker"
                  # "State timeout?"
                  # "Side changed?"
                  n223 = call "pp2_updateSideState.vi"("error in (no error)"=w292, "refnum in"=w300, "Daq config In"=w313, "State In"=w309) -> ("error out"=w293:errorcluster, "Daq config Out"=w308:T4, "State Out"=w294:T9, "State timeout"=w312:bool, "Side change"=w311:bool)  [unwired: 3 in]
                  n224 = local write "Runtime Errors"(w292) -> ()
                  n225 = local write "State info"(w294) -> ()
                  n226 = Unbundle By Name(w294) -> ("Curr State"=w286:T10)
                  n227 = case shown="\"14 Intertrial Interval\"" w286 {
                    tunnel: w314 -> [w322 w338 w353 w395 w429 w466 w488 w526 w553 w584 w596 w620]
                    tunnel: w294 -> [w325 w327 w357 w393 w433 w471 w493 w533 w550 w588 w597 w619]
                    tunnel: w312 -> [w319 _ w354 w387 w431 w469 w491 w529 w545 _ w602 _]
                    tunnel: w311 -> [_ _ w358 _ w434 w468 w490 w530 w544 _ _ _]
                    tunnel: [w324 w344 w356 w396 w432 w474 w486 w532 w551 w587 w601 w619] -> w310
                    tunnel: w308 -> [w323 w342 w352 w392 w427 w470 w492 w531 w549 w589 w600 w618]
                    tunnel: [w323 w341 w349 w391 w426 w470 w485 w531 w548 w589 w600 w618] -> w307
                    tunnel: [w322 w338 w353 w395 w429 w466 w488 w526 w553 w584 w595 w620] -> w306
                    tunnel: w305 -> [_ w339 w355 _ _ _ _ _ _ _ _ _]
                    tunnel: w304 -> [_ _ _ w397 _ _ _ _ _ _ _ _]
                    tunnel: w303 -> [_ _ _ _ w430 _ w487 _ _ _ _ _]
                    tunnel: w302 -> [_ _ w346 _ _ _ _ _ _ _ _ _]
                    tunnel: w293 -> [w317 w336 w351 w390 w425 w465 w489 w525 w547 w583 w594 w621]
                    tunnel: [w317 w335 w350 w389 w424 w465 w484 w525 w546 w583 w594 w621] -> w301
                    tunnel: w300 -> [_ w337 _ _ _ _ _ _ _ _ _ _]
                    tunnel: w299 -> [_ _ _ _ _ _ _ _ _ _ w599 w622]
                    tunnel: [FALSE FALSE FALSE FALSE FALSE FALSE FALSE FALSE FALSE FALSE w598 w622] -> w298
                    tunnel: w297 -> [_ _ _ _ _ w473 _ w528 _ w591 _ _]
                    tunnel: w296 -> [_ _ _ _ _ w472 _ w527 _ w590 _ _]
                    tunnel: [TRUE FALSE FALSE FALSE FALSE FALSE FALSE FALSE FALSE FALSE TRUE TRUE] -> w295
                    tunnel: w284 -> [_ _ w345 _ _ _ _ _ _ _ _ _]
                    frame "1 Habituation" {
                      # "Load next if timeout"
                      n228 = Wait Until Next ms Multiple(millisecond multiple=u32 1) -> ()  [unwired: 1 out]
                      n229 = call "pp2_NextState.vi"("Actually run (passthrough if off)"=w319, "New state countdown (ms)"=i64 0, "New State"=pp2_CTL_State."2 (Load Trial)", "State In"=w325) -> ("State Out"=w324:T9)  [unwired: 7 in]
                    }
                    frame "2 (Load Trial)" {
                      # "Load curr trial and apply variable shock if on.\n(will not increment)"
                      n230 = local read "Session param (dynamic)"() -> (w332:T8)
                      n231 = Unbundle By Name(w327) -> ("Curr  tr"=w326:u16)
                      n232 = control-ref of="Session list display"() -> (w328:refnum<vi>)
                      n233 = local read "Session List Hidden"() -> (w333:u8[])
                      n234 = local read "Trial Types"() -> (w334:T1[])
                      n235 = call "pp2_util_paintTableElement.vi"("Color Box"=u32 13619104, "Numeric"=w326, "Tbl Refnum"=w328) -> ()  [unwired: 9 in]
                      n236 = call "pp2_loadTrial.vi"("State Info In"=w327, "Session param (dynamic)"=w332, "Session List (Hidden variable)"=w333, "Trial Types"=w334, "Daq config In"=w342, "refnum in"=w337, "error in (no error)"=w336) -> ("State Info Out"=w343:T9, "Daq config Out"=w341:T4, "error out"=w335:errorcluster)  [unwired: 6 in]
                      n237 = call "pp2_NextState.vi"("New state countdown (ms)"=w339, "New State"=pp2_CTL_State."3 Stay Period", "State In"=w343) -> ("State Out"=w344:T9)  [unwired: 8 in]
                    }
                    frame "3 Stay Period" {
                      n238 = case shown="False" w358 {
                        tunnel: w357 -> [w367 w386]
                        tunnel: [w361 w385] -> w356
                        tunnel: w355 -> [_ w383]
                        tunnel: w354 -> [w366 _]
                        tunnel: w352 -> [w365 w382]
                        tunnel: w351 -> [w364 w381]
                        tunnel: [w363 w381] -> w350
                        tunnel: [w362 w382] -> w349
                        tunnel: w346 -> [w360 _]
                        tunnel: w345 -> [w359 _]
                        frame False {
                          n239 = case shown="True" w366 {
                            tunnel: w367 -> [w371 w380]
                            tunnel: w365 -> [w370 w378]
                            tunnel: w364 -> [w369 w377]
                            tunnel: [w369 w376] -> w363
                            tunnel: [w370 w375] -> w362
                            tunnel: [w371 w374] -> w361
                            tunnel: w360 -> [_ w373]
                            tunnel: w359 -> [_ w372]
                            frame False {
                              # "No side change, no timeout"
                              n240 = Wait Until Next ms Multiple(millisecond multiple=u32 1) -> ()  [unwired: 1 out]
                            }
                            frame True {
                              # "If stay timed out without side change, \ntrigger change to (Load audio) and play click"
                              n241 = call "pp2_NextState.vi"("New state countdown (ms)"=w372, "New State"=pp2_CTL_State."4 Load Audio/Click Delay", "State In"=w380) -> ("State Out"=w374:T9)  [unwired: 8 in]
                              n242 = call "pp2_DAQwritePlayClick.vi"("State In"=w374, "Daq config"=w378, "Pre click \n(V)"=w373, "error in (no error)"=w377) -> ("Daq config 2"=w375:T4, "error out"=w376:errorcluster)  [unwired: 5 in]
                            }
                          }
                        }
                        frame True {
                          # "If side changed during stay, reload stay period\n(will not log state change, 3 == 3)"
                          n243 = call "pp2_NextState.vi"("New state countdown (ms)"=w383, "New State"=pp2_CTL_State."3 Stay Period", "State In"=w386) -> ("State Out"=w385:T9)  [unwired: 8 in]
                        }
                      }
                    }
                    frame "4 Load Audio/Click Delay" {
                      n244 = case shown="True" w387 {
                        tunnel: w397 -> [_ w409]
                        tunnel: [w401 w408] -> w396
                        tunnel: w393 -> [w401 w407]
                        tunnel: w392 -> [w400 w405]
                        tunnel: [w400 w404] -> w391
                        tunnel: w390 -> [w399 w403]
                        tunnel: [w399 w402] -> w389
                        frame False {
                          n245 = Wait Until Next ms Multiple(millisecond multiple=u32 1) -> ()  [unwired: 1 out]
                        }
                        frame True {
                          n246 = Unbundle By Name(w407) -> ("Current Loaded Trial.Trial Type"=w410:T2)
                          n247 = call "pp2_DAQwriteAudioStimulus.vi"("State Info In"=w407, "Daq config In"=w405, "error in (no error)"=w403) -> ("State Info Out"=w406:T9, "Daq config Out"=w404:T4, "error out"=w402:errorcluster)  [unwired: 10 in]
                          n248 = case shown="\"TEST\", Default" w410 {
                            tunnel: w409 -> [w413 w417 w421]
                            tunnel: w406 -> [w412 w416 w420]
                            tunnel: [w411 w415 w419] -> w408
                            frame "GO" {
                              n249 = call "pp2_NextState.vi"("New state countdown (ms)"=w413, "New State"=pp2_CTL_State."5 GO Trial", "State In"=w412) -> ("State Out"=w411:T9)  [unwired: 8 in]
                            }
                            frame "TEST", Default {
                              n250 = call "pp2_NextState.vi"("New state countdown (ms)"=w417, "New State"=pp2_CTL_State."11 TEST Trial", "State In"=w416) -> ("State Out"=w415:T9)  [unwired: 8 in]
                            }
                            frame "NOGO" {
                              n251 = call "pp2_NextState.vi"("New state countdown (ms)"=w421, "New State"=pp2_CTL_State."8 NOGO Trial", "State In"=w420) -> ("State Out"=w419:T9)  [unwired: 8 in]
                            }
                          }
                        }
                      }
                    }
                    frame "5 GO Trial" {
                      n252 = case shown="False" w434 {
                        tunnel: w433 -> [w441 w458]
                        tunnel: [w440 w461] -> w432
                        tunnel: w431 -> [w442 _]
                        tunnel: w430 -> [w439 _]
                        tunnel: w427 -> [w438 w459]
                        tunnel: [w437 w459] -> w426
                        tunnel: w425 -> [w436 w460]
                        tunnel: [w435 w460] -> w424
                        frame False {
                          n253 = case shown="False" w442 {
                            tunnel: w441 -> [w451 w456]
                            tunnel: [w450 w454] -> w440
                            tunnel: w439 -> [_ w455]
                            tunnel: w438 -> [w448 w452]
                            tunnel: [w447 w452] -> w437
                            tunnel: w436 -> [w444 w453]
                            tunnel: [w443 w453] -> w435
                            frame False {
                              # "Just continue sound"
                              n254 = Unbundle By Name(w451) -> ("Tone countdown (ms)"=w446:i64, "Tone repeat memo"=w445:i64)
                              n255 = call "pp2_DAQplayAudio.vi"("Daq config In"=w448, "Tone countdown (ms) In"=w446, "Tone repeat memo"=w445, "error in (no error)"=w444) -> ("Daq config Out"=w447:T4, "Tone countdown (ms) Out"=w449:i64, "error out"=w443:errorcluster)  [unwired: 9 in]
                              n256 = Bundle By Name(cluster=w451, "Tone countdown (ms)"=w449) -> (w450:T9)
                            }
                            frame True {
                              # "If side not changed,\nbut timeout, miss!!"
                              n257 = call "pp2_NextState.vi"("New state countdown (ms)"=w455, "New State"=pp2_CTL_State."7 GO Timeout", "State In"=w456) -> ("State Out"=w454:T9)  [unwired: 8 in]
                            }
                          }
                        }
                        frame True {
                          # "If side changed, hit!!!"
                          n258 = call "pp2_NextState.vi"("New state countdown (ms)"=i64 0, "New State"=pp2_CTL_State."6 GO Jumped", "State In"=w458) -> ("State Out"=w461:T9)  [unwired: 8 in]
                        }
                      }
                    }
                    frame "7 GO Timeout" {
                      n259 = Or(x=w468, y=w469) -> (x .or. y?=w467:bool)
                      n260 = case shown="True" w467 {
                        tunnel: [w476 w481] -> w474
                        tunnel: w473 -> [_ w480]
                        tunnel: w472 -> [_ w479]
                        tunnel: w471 -> [w476 w477]
                        frame False {
                          # "Continue shock"
                        }
                        frame True {
                          # "If side change or timeout, escape shock"
                          # "Shock terminated here"
                          n261 = call "RandomInt64.vi"("Min"=w479, "Max"=w480) -> ("Random"=w478:i64)  [unwired: 9 in]
                          n262 = call "pp2_NextState.vi"("New state countdown (ms)"=w478, "New State"=pp2_CTL_State."14 Intertrial Interval", "State In"=w477) -> ("State Out"=w481:T9)  [unwired: 8 in]
                        }
                      }
                    }
                    frame "8 NOGO Trial" {
                      n263 = case shown="False" w490 {
                        tunnel: w493 -> [w501 w518]
                        tunnel: [w500 w522] -> w486
                        tunnel: w491 -> [w502 _]
                        tunnel: w487 -> [w499 w519]
                        tunnel: w492 -> [w498 w520]
                        tunnel: [w497 w520] -> w485
                        tunnel: w489 -> [w496 w521]
                        tunnel: [w495 w521] -> w484
                        frame False {
                          n264 = case shown="False" w502 {
                            tunnel: w501 -> [w511 w516]
                            tunnel: [w510 w515] -> w500
                            tunnel: w499 -> [_ _]
                            tunnel: w498 -> [w508 w513]
                            tunnel: [w507 w513] -> w497
                            tunnel: w496 -> [w504 w514]
                            tunnel: [w503 w514] -> w495
                            frame False {
                              # "Just continue sound"
                              n265 = Unbundle By Name(w511) -> ("Tone countdown (ms)"=w506:i64, "Tone repeat memo"=w505:i64)
                              n266 = call "pp2_DAQplayAudio.vi"("Daq config In"=w508, "Tone countdown (ms) In"=w506, "Tone repeat memo"=w505, "error in (no error)"=w504) -> ("Daq config Out"=w507:T4, "Tone countdown (ms) Out"=w509:i64, "error out"=w503:errorcluster)  [unwired: 9 in]
                              n267 = Bundle By Name(cluster=w511, "Tone countdown (ms)"=w509) -> (w510:T9)
                            }
                            frame True {
                              # "If side not changed,\nbut timeout, corr rejection"
                              n268 = call "pp2_NextState.vi"("New state countdown (ms)"=i64 0, "New State"=pp2_CTL_State."10 NOGO Timeout", "State In"=w516) -> ("State Out"=w515:T9)  [unwired: 8 in]
                            }
                          }
                        }
                        frame True {
                          # "If side changed,\nfalse alarm!!!"
                          n269 = call "pp2_NextState.vi"("New state countdown (ms)"=w519, "New State"=pp2_CTL_State."9 NOGO Jumped", "State In"=w518) -> ("State Out"=w522:T9)  [unwired: 8 in]
                        }
                      }
                    }
                    frame "9 NOGO Jumped" {
                      n270 = Or(x=w530, y=w529) -> (x .or. y?=w534:bool)
                      n271 = case shown="True" w534 {
                        tunnel: [w536 w541] -> w532
                        tunnel: w528 -> [_ w540]
                        tunnel: w527 -> [_ w539]
                        tunnel: w533 -> [w536 w537]
                        frame False {
                          # "Continue shock"
                        }
                        frame True {
                          # "If side change or timeout, escape shock"
                          n272 = call "RandomInt64.vi"("Min"=w539, "Max"=w540) -> ("Random"=w538:i64)  [unwired: 9 in]
                          n273 = call "pp2_NextState.vi"("New state countdown (ms)"=w538, "New State"=pp2_CTL_State."14 Intertrial Interval", "State In"=w537) -> ("State Out"=w541:T9)  [unwired: 8 in]
                        }
                      }
                    }
                    frame "11 TEST Trial" {
                      n274 = case shown="True" w544 {
                        tunnel: w550 -> [w559 w576]
                        tunnel: [w558 w580] -> w551
                        tunnel: w545 -> [w560 _]
                        tunnel: w549 -> [w557 w578]
                        tunnel: [w556 w578] -> w548
                        tunnel: w547 -> [w555 w579]
                        tunnel: [w554 w579] -> w546
                        frame False {
                          n275 = case shown="False" w560 {
                            tunnel: w559 -> [w569 w574]
                            tunnel: [w568 w573] -> w558
                            tunnel: w557 -> [w566 w571]
                            tunnel: [w565 w571] -> w556
                            tunnel: w555 -> [w562 w572]
                            tunnel: [w561 w572] -> w554
                            frame False {
                              # "Just continue sound"
                              n276 = Unbundle By Name(w569) -> ("Tone countdown (ms)"=w564:i64, "Tone repeat memo"=w563:i64)
                              n277 = call "pp2_DAQplayAudio.vi"("Daq config In"=w566, "Tone countdown (ms) In"=w564, "Tone repeat memo"=w563, "error in (no error)"=w562) -> ("Daq config Out"=w565:T4, "Tone countdown (ms) Out"=w567:i64, "error out"=w561:errorcluster)  [unwired: 9 in]
                              n278 = Bundle By Name(cluster=w569, "Tone countdown (ms)"=w567) -> (w568:T9)
                            }
                            frame True {
                              # "If side not changed,\nbut timeout, rejection"
                              n279 = call "pp2_NextState.vi"("New state countdown (ms)"=i64 0, "New State"=pp2_CTL_State."13 TEST Timeout", "State In"=w574) -> ("State Out"=w573:T9)  [unwired: 8 in]
                            }
                          }
                        }
                        frame True {
                          # "If side changed,\njumped"
                          n280 = call "pp2_NextState.vi"("New state countdown (ms)"=i64 0, "New State"=pp2_CTL_State."12 TEST Jumped", "State In"=w576) -> ("State Out"=w580:T9)  [unwired: 8 in]
                        }
                      }
                    }
                    frame "6 GO Jumped", "10 NOGO Timeout", "12 TEST Jumped", "13 TEST Timeout" {
                      n281 = call "RandomInt64.vi"("Min"=w590, "Max"=w591) -> ("Random"=w586:i64)  [unwired: 9 in]
                      n282 = call "pp2_NextState.vi"("New state countdown (ms)"=w586, "New State"=pp2_CTL_State."14 Intertrial Interval", "State In"=w588) -> ("State Out"=w587:T9)  [unwired: 8 in]
                    }
                    frame "14 Intertrial Interval" {
                      n283 = case shown="True" w602 {
                        tunnel: w597 -> [w610 w615]
                        tunnel: [w610 w613] -> w601
                        frame False {
                          n284 = Wait Until Next ms Multiple(millisecond multiple=u32 5) -> ()  [unwired: 1 out]
                        }
                        frame True {
                          n285 = Unbundle By Name(w615) -> ("Curr  tr"=w617:u16)
                          n286 = Increment(x=w617) -> (x+1=w616:u16)
                          n287 = Bundle By Name(cluster=w615, "Curr  tr"=w616) -> (w614:T9)
                          n288 = call "pp2_NextState.vi"("New state countdown (ms)"=i64 0, "New State"=pp2_CTL_State."2 (Load Trial)", "State In"=w614) -> ("State Out"=w613:T9)  [unwired: 8 in]
                        }
                      }
                      n289 = case shown="False" w599 {
                        selector: w599 -> [_ w608]
                        tunnel: [TRUE w608] -> w598
                        tunnel: w597 -> [w605 _]
                        tunnel: w596 -> [w604 w607]
                        tunnel: [w603 w607] -> w595
                        frame False {
                          # "Update stats once for\neach trial (first cycle 14)"
                          n290 = call "pp2_updateSessionInfo.vi"("Session info In"=w604, "State In"=w605) -> ("Session info Out"=w603:T12)  [unwired: 9 in]
                          n291 = local write "Session info"(w603) -> ()
                        }
                        frame True {
                        }
                      }
                    }
                    frame "0 NULL", "15 Done" {
                      # "\"0 Null\" Will not happen, added to fix compile error"
                    }
                  }
                  n292 = Equal?(x=w286, y=pp2_CTL_State."15 Done" ("Trial State")) -> (x = y?=w285:bool)
                  n293 = local read "stop"() -> (w291:bool)
                  n294 = Compound Arithmetic op=OR("Pause", w291, w285) -> (w289:bool)
                  n295 = And(x=w295, y=w289) -> (x .and. y?=w288:bool)
                }
                n296 = local write "Daq config"(w255) -> ()
                n297 = local write "State info"(w256) -> ()
              }
              frame #4 {
                w625 = FALSE
                # "This will stop webcam recording in\nasynchronous processs"
                # "Close log file"
                # "Clean up DAQ"
                n298 = local read "State info"() -> (w626:T9)
                n299 = Bundle By Name(cluster=w626, "Tone\nGate"=w625, "Stim"=w625, "Current DAQ DO Int"=u16 0, "Webcam recording"=w625) -> (w627:T9)
                n300 = local write "State info"(w627) -> ()
                n301 = Close File(refnum=w628) -> ()  [unwired: 1 in, 2 out]
              }
              frame #5 {
                # "Post-behavior UI adjustments"
                n302 = property on="Pause" class="Bool (strict)"("DisabledEnum"=T13."Disabled and Grayed Out" ("Disabled")) -> ()  [unwired: 2 in, 2 out]
                n303 = property on="Trial Types Control" class="TabCtl (strict)"("DisabledEnum"=T13."Enabled" ("Disabled")) -> ()  [unwired: 2 in, 2 out]
              }
            }
          }
        }
      }
    }
    frame #4 {
      w638 = FALSE ("Webcam on")
      w641 = FALSE
      w637 = T13."Enabled" ("Disabled")
      # "Clean up DAQ"
      # "Stop webcam recording"
      # "Post UI Adjustments"
      n304 = local read "State info"() -> (w639:T9)
      n305 = Bundle By Name(cluster=w639, "Webcam on"=w638, "Webcam recording"=w638) -> (w640:T9)
      n306 = local write "State info"(w640) -> ()
      n307 = property on="Daq config" class="Clust (strict)"("DisabledEnum"=w637) -> ()  [unwired: 2 in, 2 out]
      n308 = property on="Session List Control" class="TabCtl (strict)"("DisabledEnum"=w637) -> ()  [unwired: 2 in, 2 out]
      n309 = property on="Trial Types Control" class="TabCtl (strict)"("DisabledEnum"=w637) -> ()  [unwired: 2 in, 2 out]
      n310 = property on="Session param (dynamic)" class="Clust (strict)"("DisabledEnum"=w637) -> ()  [unwired: 2 in, 2 out]
      n311 = property on="State info" class="Clust (strict)"("DisabledEnum"=w637) -> ()  [unwired: 2 in, 2 out]
      n312 = property on="Session parameters" class="Clust (strict)"("DisabledEnum"=w637) -> ()  [unwired: 2 in, 2 out]
      n313 = property on="Session info" class="Clust (strict)"("DisabledEnum"=w637) -> ()  [unwired: 2 in, 2 out]
      n314 = local read "Runtime Errors"() -> (w634:errorcluster)
      n315 = local read "Daq config"() -> (w635:T4)
      n316 = local write "stop"(w641) -> ()
      n317 = local write "Pause"(w641) -> ()
      n318 = call "pp2_DAQclear.vi"("error in (no error)"=w634, "Daq config in"=w635) -> ("error out"=w631:errorcluster, "Daq config out"=w636:T4)  [unwired: 8 in]
      n319 = local write "Daq config"(w636) -> ()
      n320 = Close Reference(reference=w633, error in (no error)=w631) -> (error out=w632:errorcluster)
      n321 = local write "Runtime Errors"(w632) -> ()
    }
  }
  n322 = control-ref of="Image"() -> ()  [unwired: 1 out]
